vi "SetEvaluations.vi"(8 "Error In":errorcluster, 9 "Value":string, 10 "Label":string, 11 "reference in":refnum<class "IAuthorization.lvclass">) -> (0 "Error Out":errorcluster, 3 "reference in":refnum<class "IAuthorization.lvclass">)   [LabVIEW 2021, in "IAuthorization.lvclass"]
uses:
  IAuthorization.lvclass
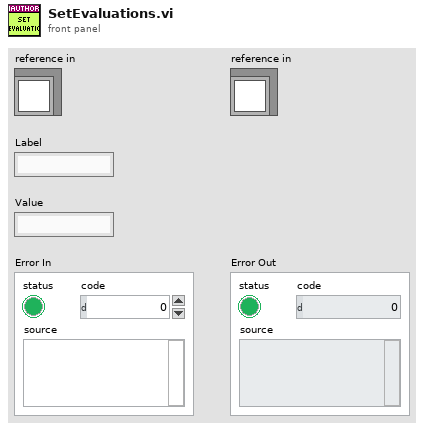
[diagram p1: front panel]
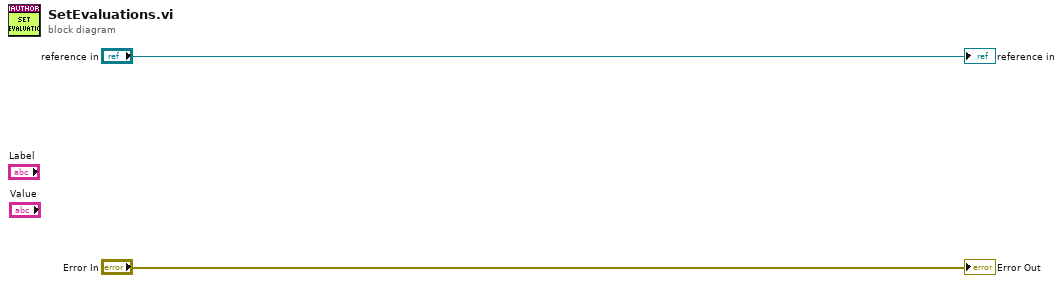
[diagram p0: block diagram]
diagram:
  "Error Out" <- "Error In"
  "reference in" <- "reference in"
